vi "Set Acyclic Frame in Trigger.vi"(8 "error in":errorcluster, 10 "acyclic frame":T1, 11 "acyclic frame trigger":T2 format="%.0x") -> (0 "error out":errorcluster, 3 "acyclic frame trigger out":T2 format="%.0x")   [LabVIEW 2020, in "AIM MIL-STD-1553 Scripting.lvlib"]
doc: "Stores the <b>acyclic frame</b> in the specified <b>acyclic frame trigger</b>. Note: Only one acyclic frame can be set for each trigger."
uses:
  AIM MIL-STD-1553 Scripting.lvlib
  <vilib>/NI VeriStand/Custom Device API/Custom Device Item Ref.ctl
  Constants.vi
  <vilib>/NI VeriStand/Custom Device API/Custom Device API.lvlib
  <vilib>/NI VeriStand/Custom Device API/Set Item Property (String Array).vi
  <vilib>/NI VeriStand/Custom Device API/Set Item Property (String).vi
  Shared/Acyclic Frame Definition.ctl
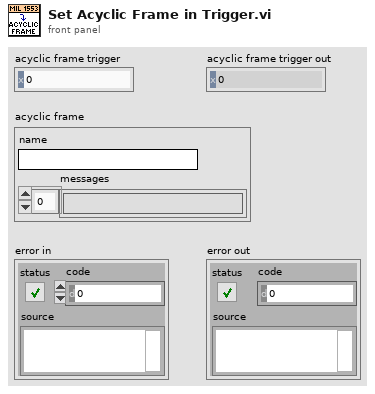
[diagram p1: front panel]
types:
  T1 = typedef "Acyclic Frame Definition.ctl" = cluster{"name":string, "messages":string[]}
  T2 = typedef "Custom Device API.lvlib/Custom Device Item Ref.ctl" = u64
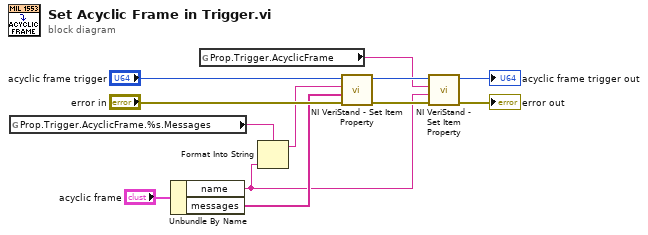
[diagram p0: block diagram]
diagram:
  n1 = global read "Constants.vi" "Prop.Trigger.AcyclicFrame.%s.Messages"() -> (w9:string)
  n2 = Unbundle By Name("acyclic frame") -> ("name"=w2:string, "messages"=w7:string[])
  n3 = global read "Constants.vi" "Prop.Trigger.AcyclicFrame"() -> (w1:string)
  n4 = Format Into String(format string=w9, w2) -> (resulting string=w8:string)  [unwired: 2 in, 1 out]
  n5 = call-poly <vilib>:"NI VeriStand - Set Item Property.vi"("error in (no error)"="error in", "Value"=w7, "Property Name"=w8, "Item Ref in"="acyclic frame trigger") -> ("error out"=w5:errorcluster, "Item Ref out"=w6:T2)  [unwired: 5 in, 1 out]
  n6 = call-poly <vilib>:"NI VeriStand - Set Item Property.vi"("error in (no error)"=w5, "Value"=w2, "Property Name"=w1, "Item Ref in"=w6) -> ("error out"=→"error out":errorcluster, "Item Ref out"=→"acyclic frame trigger out":T2)  [unwired: 5 in, 1 out]
